vi "SwerveDriveSafetyError.vi"(0 "SwerveDriveDevRef":T1={"DevStatus"={"status"=FALSE, "code"=0, "source"=""}, "TurnMotors[]"=[], "Square Inputs"=FALSE, "Max Output"=1.0, "DriveMotors[]"=[], "WheelOffset[]"=[], "SwerveSensors[]"=[], "RobotSize"={"Width"=[], "Length"=[], "Center"=[]}}) -> ()   [LabVIEW 2019, in "Swerve Drive.lvlib"]
doc: "This subVI does two things:\n1. It builds up output specific information to help locate the problem.\n2. It calls the FRC Build Error, so all the information gets passed to the Driver Station."
uses:
  Swerve Drive.lvlib
  SwerveDriveDevRef.ctl
  <vilib>/Rock Robotics/WPI/MotorControl/WPI_MotorControlDeviceRef.ctl
  <vilib>/Rock Robotics/WPI/MotorControl/WPI_MotorControlType.ctl
  <vilib>/Rock Robotics/SystemInterfaces/DIO/FPGA_DIOPWMChannel.ctl
  <vilib>/Rock Robotics/WPI/PWM/WPI_PWMDeadband.ctl
  <vilib>/Rock Robotics/SystemInterfaces/DIO/FPGA_DIOChannel.ctl
  <vilib>/Rock Robotics/SystemInterfaces/AI/FPGA_AIChannel.ctl
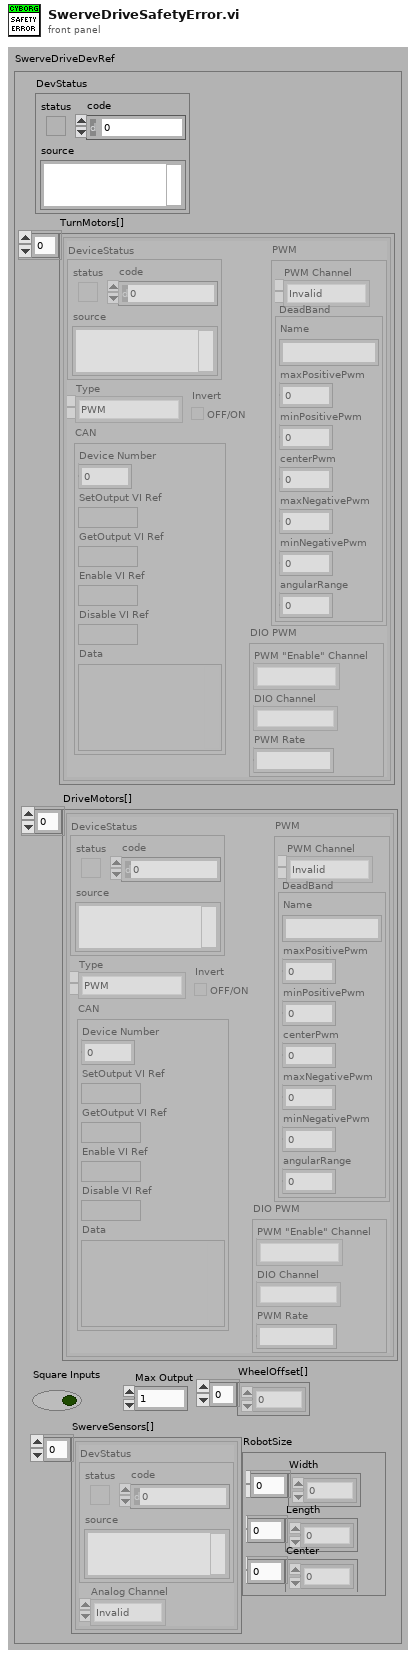
[diagram p1: front panel]
types:
  T1 = typedef "Swerve Drive.lvlib/SwerveDriveDevRef.ctl" = cluster{"DevStatus":errorcluster, "TurnMotors[]":T2[], "Square Inputs":bool, "Max Output":dbl, "DriveMotors[]":T2[], "WheelOffset[]":dbl[], "SwerveSensors[]":cluster{"DevStatus":errorcluster, "Analog Channel":T7}[], "RobotSize":cluster{"Width":dbl[], "Length":dbl[], "Center":dbl[]}}
  T2 = typedef "WPI_MotorControlDeviceRef.ctl" = cluster{"DeviceStatus":errorcluster, "Type":T3, "PWM":cluster{"PWM Channel":T4, "DeadBand":T5}, "CAN":cluster{"Device Number":u8, "SetOutput VI Ref":variant, "GetOutput VI Ref":variant, "Enable VI Ref":variant, "Disable VI Ref":variant, "Data":variant}, "Invert":bool, "DIO PWM":cluster{"PWM \"Enable\" Channel":T4, "DIOChannel":T6, "PWM Rate":dbl}}
  T3 = typedef "WPI_MotorControlType.ctl" = enum16{"PWM", "CAN", "DIO PWM"}
  T4 = typedef "FPGA_DIOPWMChannel.ctl" = enum8{"PWM 0", "PWM 1", "PWM 2", "PWM 3", "PWM 4", "PWM 5", "PWM 6", "PWM 7", "PWM 8", "PWM 9", "PWM MXP 0", "PWM MXP 1", "PWM MXP 2", "PWM MXP 3", "PWM MXP 4", "PWM MXP 5", "PWM MXP 6", "PWM MXP 7", "PWM MXP 8", "PWM MXP 9", "Invalid"}
  T5 = typedef "WPI_PWMDeadband.ctl" = cluster{"Name":string, "maxPositivePwm":i32, "minPositivePwm":i32, "centerPwm":i32, "maxNegativePwm":i32, "minNegativePwm":i32, "angularRange":u16}
  T6 = typedef "FPGA_DIOChannel.ctl" = enum8{"DIO 0", "DIO 1", "DIO 2", "DIO 3", "DIO 4", "DIO 5", "DIO 6", "DIO 7", "DIO 8", "DIO 9", "DIO MXP 0", "DIO MXP 1", "DIO MXP 2", "DIO MXP 3", "DIO MXP 4", "DIO MXP 5", "DIO MXP 6", "DIO MXP 7", "DIO MXP 8", "DIO MXP 9", "DIO MXP 10", "DIO MXP 11", "DIO MXP 12", "DIO MXP 13", "DIO MXP 14", "DIO MXP 15", "SPI Port CS1", "SPI Port CS2", "SPI Port CS3", "SPI Port MISO", "SPI Port MOSI", "Invalid"}
  T7 = typedef "FPGA_AIChannel.ctl" = enum8{"AI 0", "AI 1", "AI 2", "AI 3", "AI MXP 0", "AI MXP 1", "AI MXP 2", "AI MXP 3", "Invalid"}
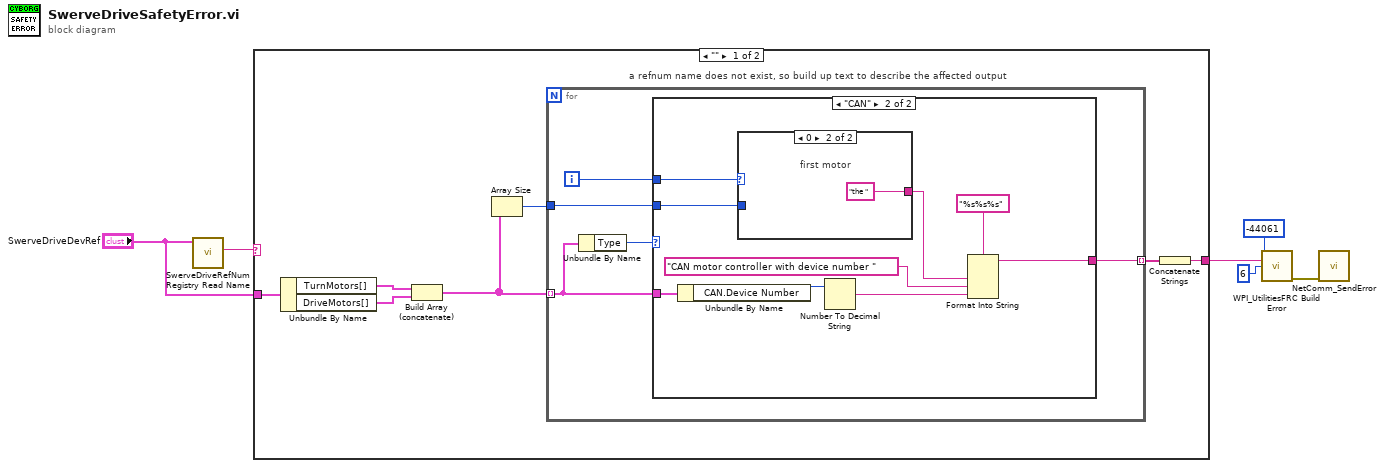
[diagram p0: block diagram]
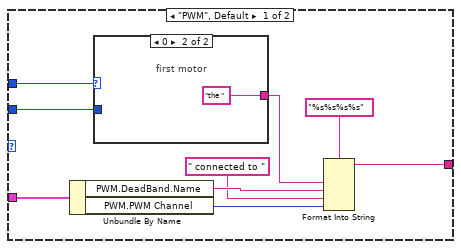
[diagram p2: hidden frame]
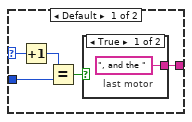
[diagram p3: hidden frame]
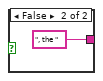
[diagram p4: hidden frame]
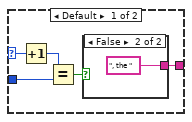
[diagram p5: hidden frame]
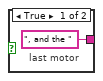
[diagram p6: hidden frame]
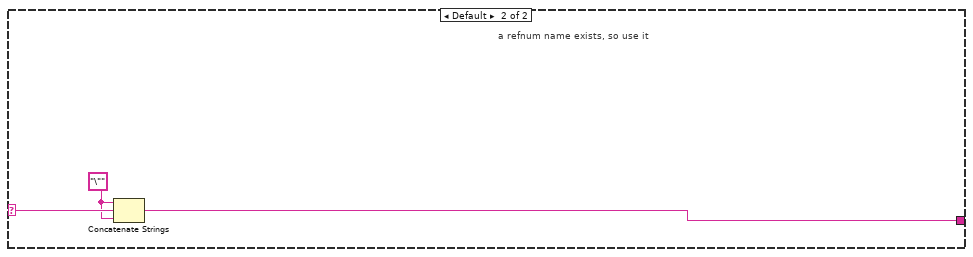
[diagram p7: hidden frame]
diagram:
  n1 = call "SwerveDriveRefNum Registry Read Name.vi"("SwerveDriveDevRef"="SwerveDriveDevRef") -> ("refnum name"=w4:string)  [unwired: 8 in, 2 out]
  n2 = case shown="\"\"" w4 {
    selector: w4 -> [_ w55]
    tunnel: [w9 w54] -> w3
    tunnel: "SwerveDriveDevRef" -> [w13 _]
    frame "" {
      # "a refnum name does not exist, so build up text to describe the affected output"
      n3 = Unbundle By Name(w13) -> ("TurnMotors[]"=w11:T2[], "DriveMotors[]"=w7:T2[])
      n4 = Build Array (concatenate)(w11, w7) -> (w8:T2[])
      n5 = Array Size(array=w8) -> (size(s)=w10:i32)
      n6 = for {
        tunnel: w8 -> [w15] mode=indexing
        tunnel: [w18] -> w12 mode=indexing
        tunnel: w10 -> [w16]
        i -> [w17]
        n7 = Unbundle By Name(w15) -> ("Type"=w14:T3)
        n8 = case shown="\"CAN\"" w14 {
          tunnel: [w23 w43] -> w18
          tunnel: w17 -> [w22 w42]
          tunnel: w16 -> [w21 w41]
          tunnel: w15 -> [w19 w39]
          frame "PWM", Default {
            n9 = Unbundle By Name(w19) -> ("PWM.DeadBand.Name"=w26:string, "PWM.PWM Channel"=w24:T4)
            n10 = case shown="0" w22 {
              selector: w22 -> [w32 _]
              tunnel: w21 -> [w29 _]
              tunnel: [w28 "the " ("format string")] -> w20
              frame Default {
                n11 = Increment(x=w32) -> (x+1=w30:i32)
                n12 = Equal?(x=w30, y=w29) -> (x = y?=w31:bool)
                n13 = case shown="True" w31 {
                  tunnel: [", and the " ("format string") ", the " ("format string")] -> w28
                  frame True {
                    # "last motor"
                  }
                  frame False {
                  }
                }
              }
              frame 0 {
                # "first motor"
              }
            }
            n14 = Format Into String(format string="%s%s%s%s", w20, w26, " connected to " ("format string"), w24) -> (resulting string=w23:string)  [unwired: 2 in, 1 out]
          }
          frame "CAN" {
            n15 = Unbundle By Name(w39) -> ("CAN.Device Number"=w37:u8)
            n16 = case shown="0" w42 {
              selector: w42 -> [w49 _]
              tunnel: w41 -> [w46 _]
              tunnel: [w45 "the " ("format string")] -> w40
              frame Default {
                n17 = Increment(x=w49) -> (x+1=w47:i32)
                n18 = Equal?(x=w47, y=w46) -> (x = y?=w48:bool)
                n19 = case shown="False" w48 {
                  tunnel: [", and the " ("format string") ", the " ("format string")] -> w45
                  frame True {
                    # "last motor"
                  }
                  frame False {
                  }
                }
              }
              frame 0 {
                # "first motor"
              }
            }
            n20 = Number To Decimal String(number=w37) -> (decimal integer string=w38:string)  [unwired: 1 out]
            n21 = Format Into String(format string="%s%s%s", w40, "CAN motor controller with device number " ("format string"), w38) -> (resulting string=w43:string)  [unwired: 2 in, 1 out]
          }
        }
      }
      n22 = Concatenate Strings(w12) -> (w9:string)
    }
    frame Default {
      w53 = "\"" ("string")
      # "a refnum name exists, so use it"
      n23 = Concatenate Strings(w53, w55, w53) -> (w54:string)
    }
  }
  n24 = call <vilib>:"WPI_UtilitiesFRC Build Error.vi"("error code"=-44061 ("code"), "extra error text"=w3, "chain levels to remove (1)"=6) -> ("error out"=w2:errorcluster)  [unwired: 3 in, 9 out]
  n25 = call <vilib>:"NetComm_SendError.vi"("error in (no error)"=w2) -> ()  [unwired: 11 in]
